vi "Insert File Content.vi"(8 "error in":errorcluster, 11 "Report Viewer in":refnum<class "Report Viewer.lvclass">) -> (0 "error out":errorcluster, 3 "Report Viewer out":refnum<class "Report Viewer.lvclass">)   [LabVIEW 2023, in "Report Viewer.lvlib" / "Report Viewer.lvclass"]
uses:
  Library/Report Viewer.lvclass
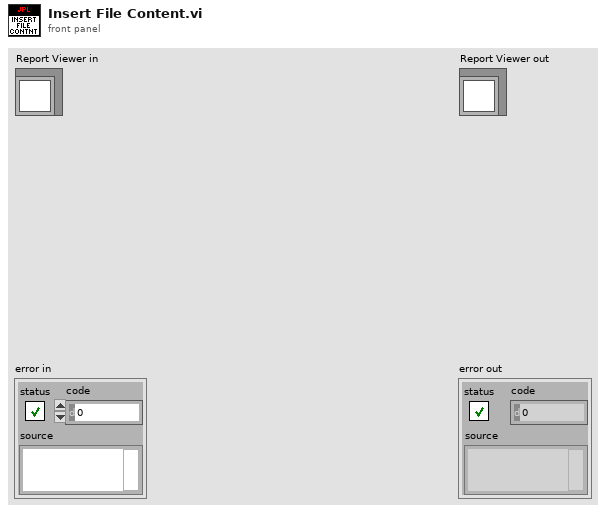
[diagram p1: front panel]
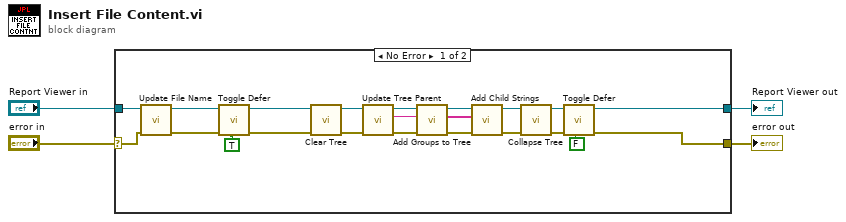
[diagram p0: block diagram]
diagram:
  n1 = case shown="No Error" "error in" {
    selector: "error in" -> [w17 w28]
    tunnel: [w7 w28] -> w3
    tunnel: [w6 w27] -> w1
    tunnel: "Report Viewer in" -> [w18 w27]
    frame No Error {
      n2 = call "Update File Name.vi"("error in"=w17, "Report Viewer in"=w18) -> ("error out"=w15:errorcluster, "Report Viewer out"=w16:refnum<class "Report Viewer.lvclass">)  [unwired: 8 in]
      n3 = call "Toggle Defer.vi"("Defer"=TRUE, "error in"=w15, "Report Viewer in"=w16) -> ("error out"=w14:errorcluster, "Report Viewer out"=w13:refnum<class "Report Viewer.lvclass">)  [unwired: 7 in]
      n4 = call "Clear Tree.vi"("error in"=w14, "Report Viewer in"=w13) -> ("error out"=w20:errorcluster, "Report Viewer out"=w21:refnum<class "Report Viewer.lvclass">)  [unwired: 8 in]
      n5 = call "Update Tree Parent.vi"("error in"=w20, "Report Viewer in"=w21) -> ("error out"=w24:errorcluster, "Tree Items Parent"=w25:string, "Report Viewer out"=w26:refnum<class "Report Viewer.lvclass">)  [unwired: 7 in]
      n6 = call "Add Groups to Tree.vi"("error in"=w24, "Tree Items Parent"=w25, "Report Viewer in"=w26) -> ("error out"=w22:errorcluster, "Group_Based_Items"=w19:string[], "Report Viewer out"=w23:refnum<class "Report Viewer.lvclass">)  [unwired: 6 in]
      n7 = call "Add Child Strings.vi"("error in"=w22, "Group_Based_Items"=w19, "Report Viewer in"=w23) -> ("error out"=w11:errorcluster, "Report Viewer out"=w10:refnum<class "Report Viewer.lvclass">)  [unwired: 7 in]
      n8 = call "Collapse Tree.vi"("error in"=w11, "Report Viewer in"=w10) -> ("error out"=w8:errorcluster, "Report Viewer out"=w9:refnum<class "Report Viewer.lvclass">)  [unwired: 8 in]
      n9 = call "Toggle Defer.vi"("Defer"=FALSE, "error in"=w8, "Report Viewer in"=w9) -> ("error out"=w7:errorcluster, "Report Viewer out"=w6:refnum<class "Report Viewer.lvclass">)  [unwired: 7 in]
    }
    frame Error {
    }
  }
  "error out" <- w3
  "Report Viewer out" <- w1
